vi "Initialise.vi"   [LabVIEW 2021, in "d18.lvlib"]
uses:
  d18.lvlib
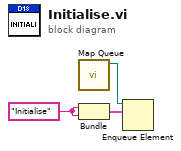
[diagram p0: block diagram]
diagram:
  w1 = "Initialise"
  n1 = call "Map Queue.vi"() -> ("Queue out"=w2:refnum<queue>)  [unwired: 11 in]
  n2 = Bundle(w1, w1) -> (w3:cluster{string, string})  [unwired: 1 in]
  n3 = Enqueue Element(queue=w2, element=w3) -> ()  [unwired: 2 in, 3 out]
